vi "home.vi"(6 "error in":errorcluster, 8 "Axis in":i32=1, 9 "VISA Handle in":refnum<visa-resource-name>) -> (0 "error out":errorcluster, 2 "Axis out":i32=1, 3 "VISA Handle out":refnum<visa-resource-name>, 4 "TimeoutFlag":bool)   [LabVIEW 2018]
doc: "This VI starts the execution of the HOME search sequence as defined by the set home type command."
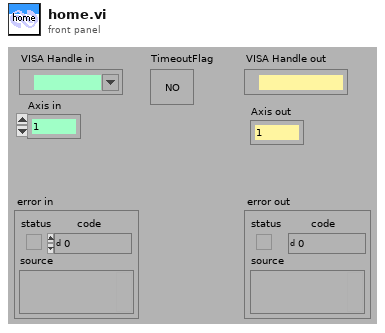
[diagram p1: front panel]
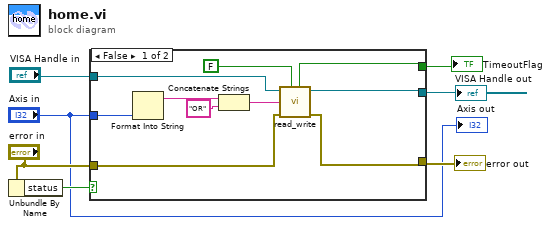
[diagram p0: block diagram]
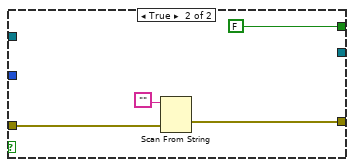
[diagram p2: hidden frame]
diagram:
  n1 = Unbundle By Name("error in") -> ("status"=w5:bool)
  n2 = case shown="False" w5 {
    tunnel: [w14 _] -> w7
    tunnel: [w13 w20] -> w6
    tunnel: "error in" -> [w15 w20]
    tunnel: [w12 FALSE ("TimeoutFlag")] -> w3
    tunnel: "Axis in" -> [w8 _]
    tunnel: "VISA Handle in" -> [w9 _]
    frame False {
      n3 = Format Into String(w8) -> (resulting string=w10:string)  [unwired: 3 in, 1 out]
      n4 = Concatenate Strings(w10, "OR" ("string")) -> (w16:string)
      n5 = call "read_write.vi"("Query?"=FALSE, "error in"=w15, "Command"=w16, "VISA handle in"=w9) -> ("error out"=w13:errorcluster, "VISA handle out"=w14:refnum<visa-resource-name>, "TimeoutFlag"=w12:bool)  [unwired: 2 in, 1 out]
    }
    frame True {
      n6 = Scan From String(input string="") -> ()  [unwired: 5 in, 3 out]
    }
  }
  "VISA Handle out" <- w7
  "error out" <- w6
  "TimeoutFlag" <- w3
  "Axis out" <- "Axis in"
